vi "Receive.vi"(8 "error in (no error)":errorcluster, 9 "timeout in ms (0)":i32, 11 "Local Queues in":T1) -> (0 "error out":errorcluster, 1 "Timeout?":bool, 2 "Packet Received":u8[](array[numeric]), 3 "Local Queues out":T1)   [LabVIEW 2020, in "Communication VIs.lvlib" / "Local.lvlib"]
uses:
  Local.lvlib
  Local Queues.ctl
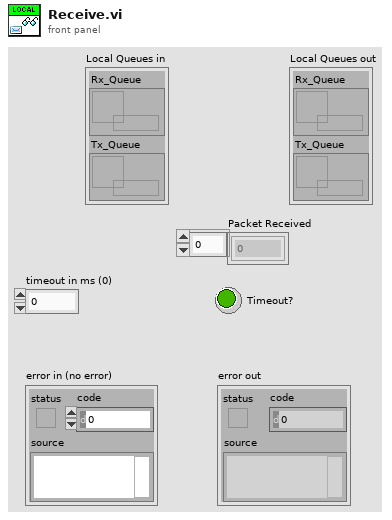
[diagram p1: front panel]
types:
  T1 = typedef "Communication VIs.lvlib/Local.lvlib/Local Queues.ctl" = cluster{"Rx_Queue":refnum<queue>, "Tx_Queue":refnum<queue>}
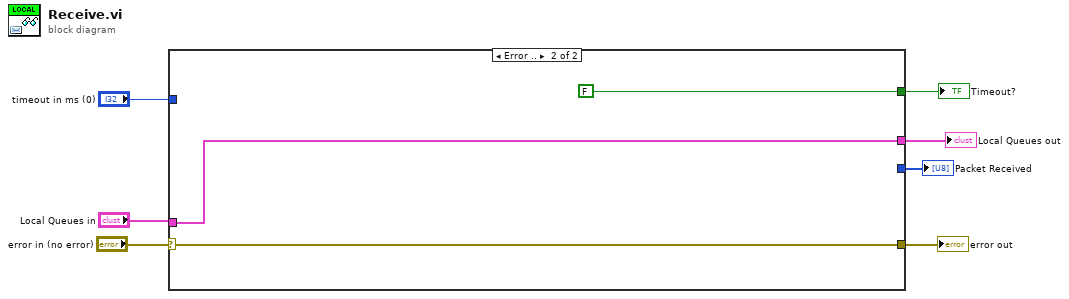
[diagram p0: block diagram]
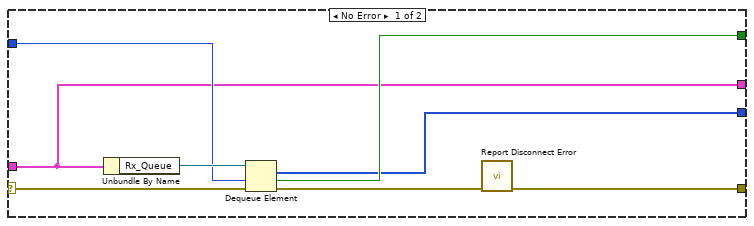
[diagram p2: hidden frame]
diagram:
  n1 = case shown="Error .." "error in (no error)" {
    selector: "error in (no error)" -> [w11 w16]
    tunnel: "timeout in ms (0)" -> [w13 _]
    tunnel: [w9 w16] -> w6
    tunnel: [w14 FALSE ("timed out?")] -> w5
    tunnel: "Local Queues in" -> [w12 w17]
    tunnel: [w12 w17] -> w2
    tunnel: [w8 _] -> w1
    frame No Error {
      n2 = Unbundle By Name(w12) -> ("Rx_Queue"=w15:refnum<queue>)
      n3 = Dequeue Element(queue=w15, timeout in ms (-1)=w13, error in (no error)=w11) -> (element=w8:u8[], timed out?=w14:bool, error out=w10:errorcluster)  [unwired: 1 out]
      n4 = call "Report Disconnect Error.vi"("error in (no error)"=w10) -> ("error out"=w9:errorcluster)  [unwired: 10 in]
    }
    frame Error {
    }
  }
  "error out" <- w6
  "Timeout?" <- w5
  "Local Queues out" <- w2
  "Packet Received" <- w1
